vi "marconi simple.vi"(9 "Frequency (MHz)":dbl=10.0 caption="Frequency  (MHz)", 10 "RF Level (dBm)":dbl=-10.0, 11 "resource name":refnum<visa-resource-name>="GPIB0::7::INSTR") -> ()   [LabVIEW 2019]
panel:
  out "error out":errorcluster
  out "RF Level":dbl=-20.0
  out "Frequency":dbl=10000000.0
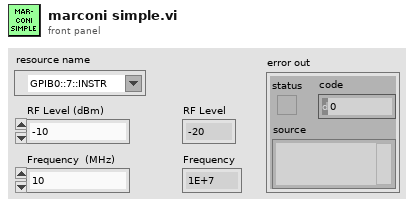
[diagram p1: front panel]
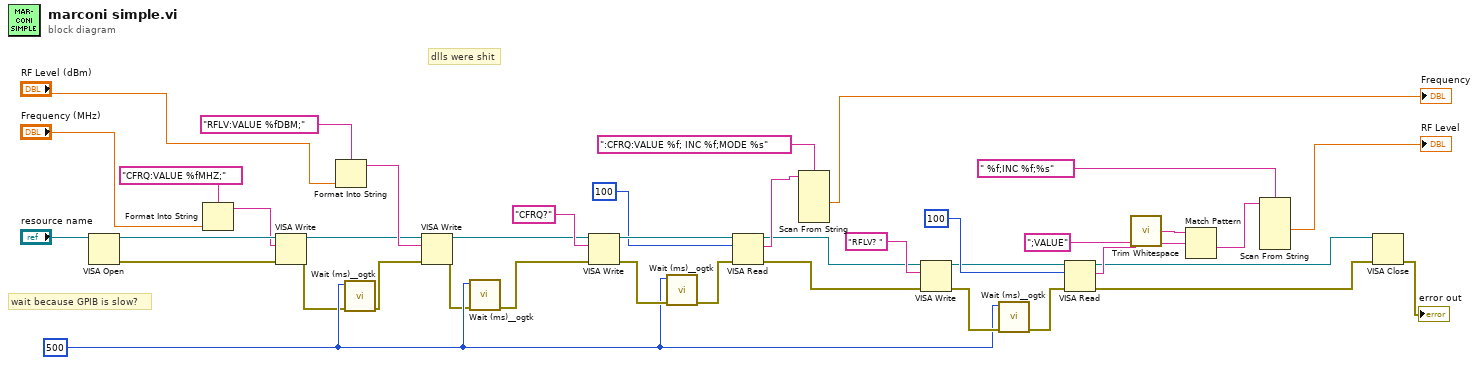
[diagram p0: block diagram]
diagram:
  w14 = u32 500 ("milliseconds to wait")
  # "dlls were shit"
  # "wait because GPIB is slow?"
  n1 = VISA Open(VISA resource name="resource name") -> (VISA resource name=w10:refnum<visa-resource-name>, error out=w35:errorcluster)  [unwired: 4 in]
  n2 = Format Into String(format string="CFRQ:VALUE %fMHZ;", "Frequency (MHz)") -> (resulting string=w8:string)  [unwired: 2 in, 1 out]
  n3 = VISA Write(VISA resource name=w10, write buffer=w8, error in (no error)=w35) -> (VISA resource name out=w5:refnum<visa-resource-name>, error out=w4:errorcluster)  [unwired: 1 out]
  n4 = Format Into String(format string="RFLV:VALUE %fDBM;", "RF Level (dBm)") -> (resulting string=w6:string)  [unwired: 2 in, 1 out]
  n5 = call <userlib>:"Wait (ms)__ogtk.vi"("error in (no error)"=w4, "milliseconds to wait"=w14) -> ("error out"=w1:errorcluster)  [unwired: 8 in, 1 out]
  n6 = VISA Write(VISA resource name=w5, write buffer=w6, error in (no error)=w1) -> (VISA resource name out=w2:refnum<visa-resource-name>, error out=w3:errorcluster)  [unwired: 1 out]
  n7 = call <userlib>:"Wait (ms)__ogtk.vi"("error in (no error)"=w3, "milliseconds to wait"=w14) -> ("error out"=w32:errorcluster)  [unwired: 8 in, 1 out]
  n8 = VISA Write(VISA resource name=w2, write buffer="CFRQ?", error in (no error)=w32) -> (VISA resource name out=w34:refnum<visa-resource-name>, error out=w29:errorcluster)  [unwired: 1 out]
  n9 = call <userlib>:"Wait (ms)__ogtk.vi"("error in (no error)"=w29, "milliseconds to wait"=w14) -> ("error out"=w28:errorcluster)  [unwired: 8 in, 1 out]
  n10 = VISA Read(VISA resource name=w34, byte count=u32 100, error in (no error)=w28) -> (VISA resource name out=w18:refnum<visa-resource-name>, read buffer=w27:string, error out=w17:errorcluster)  [unwired: 1 out]
  n11 = Scan From String(format string=":CFRQ:VALUE %f; INC %f;MODE %s", input string=w27) -> (output 1=→"Frequency":dbl)  [unwired: 7 in, 3 out]
  n12 = VISA Write(VISA resource name=w18, write buffer="RFLV? ", error in (no error)=w17) -> (VISA resource name out=w19:refnum<visa-resource-name>, error out=w22:errorcluster)  [unwired: 1 out]
  n13 = call <userlib>:"Wait (ms)__ogtk.vi"("error in (no error)"=w22, "milliseconds to wait"=w14) -> ("error out"=w23:errorcluster)  [unwired: 8 in, 1 out]
  n14 = VISA Read(VISA resource name=w19, byte count=u32 100, error in (no error)=w23) -> (VISA resource name out=w16:refnum<visa-resource-name>, read buffer=w24:string, error out=w15:errorcluster)  [unwired: 1 out]
  n15 = call <vilib>:"Trim Whitespace.vi"("string"=w24) -> ("trimmed string"=w12:string)  [unwired: 1 in]
  n16 = Match Pattern(string=w12, regular expression=";VALUE" ("format string")) -> (after substring=w11:string)  [unwired: 1 in, 3 out]
  n17 = Scan From String(format string=" %f;INC %f;%s", input string=w11) -> (output 1=→"RF Level":dbl)  [unwired: 7 in, 3 out]
  n18 = VISA Close(VISA resource name=w16, error in (no error)=w15) -> (error out=→"error out":errorcluster)
